vi "PicoScopeospaExampleStreamingQueue.vi"() -> ()   [LabVIEW 2010]
doc: "psospa Streaming example filling a single set of channel buffers at a time with LabVIEW queues."
uses:
  shared/PicoBuffers.ctl
  <vilib>/Waveform/DWDTOps.llb/DWDT Analog to Digital.vi
  PicoScopepsospaLib/PicoScopeospaDigitalChannelSettings.ctl
  PicoScopepsospaLib/PicoScopeospaAnalogChannelSettings.ctl
  shared/Buffer and Transfer Settings.ctl
panel:
  out "overflow":i16 format="%06b"
  in  "Channels":T1={"Channel A Settings "={"Enabled"=TRUE, "Coupling"=1, "Range"=8, "Analogue Offset"=0.0, "BandWidth"=0, "PROBE_RANGE_INFO"=0}, "Channel B Settings "={"Enabled"=FALSE, "Coupling"=1, "Range"=8, "Analogue Offset"=0.0, "BandWidth"=0, "PROBE_RANGE_INFO"=0}, "Channel C Settings "={"Enabled"=FALSE, "Coupling"=1, "Range"=8, "Analogue Offset"=0.0, "BandWidth"=0, "PROBE_RANGE_INFO"=0}, "Channel D Settings "={"Enabled"=FALSE, "Coupling"=1, "Range"=8, "Analogue Offset"=0.0, "BandWidth"=0, "PROBE_RANGE_INFO"=0}, "Channel E Settings "={"Enabled"=FALSE, "Coupling"=50, "Range"=5, "Analogue Offset"=0.0, "BandWidth"=0, "PROBE_RANGE_INFO"=0}, "Channel F Settings "={"Enabled"=FALSE, "Coupling"=50, "Range"=5, "Analogue Offset"=0.0, "BandWidth"=0, "PROBE_RANGE_INFO"=0}, "Channel G Settings "={"Enabled"=FALSE, "Coupling"=50, "Range"=5, "Analogue Offset"=0.0, "BandWidth"=0, "PROBE_RANGE_INFO"=0}, "Channel H Settings "={"Enabled"=FALSE, "Coupling"=50, "Range"=5, "Analogue Offset"=0.0, "BandWidth"=0, "PROBE_RANGE_INFO"=0}} {"Channel H Settings"."PROBE_RANGE_INFO" items=["PROBE_NONE_NV"=0, "X1_PROBE_NV"=1, "X10_PROBE_NV"=10]; "Channel H Settings"."BandWidth" items=["Full"=0, "100kHz"=100000, "20kHz"=200000, "1MHz"=1000000, "20MHz"=20000000, "25MHz"=25000000, "50MHz"=50000000, "200MHz"=200000000, "250MHz"=250000000, "500MHz"=500000000]; "Channel H Settings"."Range" items=["10mV"=0, "20mV"=1, "50mV"=2, "100mV"=3, "200mV"=4, "500mV"=5, "1V"=6, "2V"=7, "5V"=8, "10V"=9, "20V"=10, "50V"=11, "100V"=12, "200V"=13, "x10_Probe_100mV"=32, "x10_Probe_200mV"=33, "x10_Probe_500mV"=34, "x10_Probe_1V"=35, "x10_Probe_2V"=36, "x10_Probe_5V"=37, "x10_Probe_10V"=38, "x10_Probe_20V"=39, "x10_Probe_50V"=40, "x10_Probe_100V"=41, "x10_Probe_200V"=42, "x10_Probe_500V"=43, "CURRENT_CLAMP_60A_2A"=10500, "CURRENT_CLAMP_60A_5A"=10501, "CURRENT_CLAMP_60A_10A"=10502, "CURRENT_CLAMP_60A_20A"=10503, "CURRENT_CLAMP_60A_50A"=10504, "CURRENT_CLAMP_60A_60A"=10505, "CURRENT_CLAMP_60A_V2_0_5A"=10600, "CURRENT_CLAMP_60A_V2_1A"=10601, "CURRENT_CLAMP_60A_V2_2A"=10602, "CURRENT_CLAMP_60A_V2_5A"=10603, "CURRENT_CLAMP_60A_V2_10A"=10604, "CURRENT_CLAMP_60A_V2_20A"=10605, "CURRENT_CLAMP_60A_V2_50A"=10606, "CURRENT_CLAMP_60A_V2_60A"=10607, "RESISTANCE_LEAD_NEG5_TO_20OHM"=7000, "RESISTANCE_LEAD_NEG50_TO_200OHM"=7001, "RESISTANCE_LEAD_NEG500_TO_2KOHM"=7002, "RESISTANCE_LEAD_NEG5K_TO_20KOHM"=7003, "RESISTANCE_LEAD_NEG50K_TO_LEAD_200KOHM"=7004, "RESISTANCE_LEAD_NEG500K_TO_LEAD_2MOHM"=7005, "RESISTANCE_LEAD_DIODE_TEST"=7006, "HT_NEG3_TO_5KV"=8950, "HT_NEG3_TO_10KV"=8951, "HT_NEG5_TO_20KV"=8952, "HT_NEG5_TO_50KV"=8953, "HT_NEG5_TO_100KV"=8954, "HT_NEG3_TO_5KV_INVERTED"=8955, "HT_NEG3_TO_10KV_INVERTED"=8956, "HT_NEG5_TO_20KV_INVERTED"=8957, "HT_NEG5_TO_50KV_INVERTED"=8958, "HT_NEG5_TO_100KV_INVERTED"=8959, "TEMPERATURE_NEG50_TO_150DEGC"=9000, "PRESSURE_SENSOR_-100k-150k_PASCALS"=9100, "PRESSURE_SENSOR_-100k_TO_400k_PASCALS"=9101, "PRESSURE_SENSOR_-200k_TO_800k_PASCALS"=9102, "PRESSURE_SENSOR_-400k_TO_1600k_PASCALS"=9103, "PRESSURE_SENSOR_-400k_TO_3400k_PASCALS"=9104, "PRESSURE_SENSOR_-150k_TO_1350k_PASCALS"=9105]; "Channel H Settings"."Coupling" items=["AC"=0, "DC 1M Ohm"=1, "DC 50 Ohm"=50]; "Channel G Settings"."PROBE_RANGE_INFO" items=["PROBE_NONE_NV"=0, "X1_PROBE_NV"=1, "X10_PROBE_NV"=10]; "Channel G Settings"."BandWidth" items=["Full"=0, "100kHz"=100000, "20kHz"=200000, "1MHz"=1000000, "20MHz"=20000000, "25MHz"=25000000, "50MHz"=50000000, "200MHz"=200000000, "250MHz"=250000000, "500MHz"=500000000]; "Channel G Settings"."Range" items=["10mV"=0, "20mV"=1, "50mV"=2, "100mV"=3, "200mV"=4, "500mV"=5, "1V"=6, "2V"=7, "5V"=8, "10V"=9, "20V"=10, "50V"=11, "100V"=12, "200V"=13, "x10_Probe_100mV"=32, "x10_Probe_200mV"=33, "x10_Probe_500mV"=34, "x10_Probe_1V"=35, "x10_Probe_2V"=36, "x10_Probe_5V"=37, "x10_Probe_10V"=38, "x10_Probe_20V"=39, "x10_Probe_50V"=40, "x10_Probe_100V"=41, "x10_Probe_200V"=42, "x10_Probe_500V"=43, "CURRENT_CLAMP_60A_2A"=10500, "CURRENT_CLAMP_60A_5A"=10501, "CURRENT_CLAMP_60A_10A"=10502, "CURRENT_CLAMP_60A_20A"=10503, "CURRENT_CLAMP_60A_50A"=10504, "CURRENT_CLAMP_60A_60A"=10505, "CURRENT_CLAMP_60A_V2_0_5A"=10600, "CURRENT_CLAMP_60A_V2_1A"=10601, "CURRENT_CLAMP_60A_V2_2A"=10602, "CURRENT_CLAMP_60A_V2_5A"=10603, "CURRENT_CLAMP_60A_V2_10A"=10604, "CURRENT_CLAMP_60A_V2_20A"=10605, "CURRENT_CLAMP_60A_V2_50A"=10606, "CURRENT_CLAMP_60A_V2_60A"=10607, "RESISTANCE_LEAD_NEG5_TO_20OHM"=7000, "RESISTANCE_LEAD_NEG50_TO_200OHM"=7001, "RESISTANCE_LEAD_NEG500_TO_2KOHM"=7002, "RESISTANCE_LEAD_NEG5K_TO_20KOHM"=7003, "RESISTANCE_LEAD_NEG50K_TO_LEAD_200KOHM"=7004, "RESISTANCE_LEAD_NEG500K_TO_LEAD_2MOHM"=7005, "RESISTANCE_LEAD_DIODE_TEST"=7006, "HT_NEG3_TO_5KV"=8950, "HT_NEG3_TO_10KV"=8951, "HT_NEG5_TO_20KV"=8952, "HT_NEG5_TO_50KV"=8953, "HT_NEG5_TO_100KV"=8954, "HT_NEG3_TO_5KV_INVERTED"=8955, "HT_NEG3_TO_10KV_INVERTED"=8956, "HT_NEG5_TO_20KV_INVERTED"=8957, "HT_NEG5_TO_50KV_INVERTED"=8958, "HT_NEG5_TO_100KV_INVERTED"=8959, "TEMPERATURE_NEG50_TO_150DEGC"=9000, "PRESSURE_SENSOR_-100k-150k_PASCALS"=9100, "PRESSURE_SENSOR_-100k_TO_400k_PASCALS"=9101, "PRESSURE_SENSOR_-200k_TO_800k_PASCALS"=9102, "PRESSURE_SENSOR_-400k_TO_1600k_PASCALS"=9103, "PRESSURE_SENSOR_-400k_TO_3400k_PASCALS"=9104, "PRESSURE_SENSOR_-150k_TO_1350k_PASCALS"=9105]; "Channel G Settings"."Coupling" items=["AC"=0, "DC 1M Ohm"=1, "DC 50 Ohm"=50]; "Channel F Settings"."PROBE_RANGE_INFO" items=["PROBE_NONE_NV"=0, "X1_PROBE_NV"=1, "X10_PROBE_NV"=10]; "Channel F Settings"."BandWidth" items=["Full"=0, "100kHz"=100000, "20kHz"=200000, "1MHz"=1000000, "20MHz"=20000000, "25MHz"=25000000, "50MHz"=50000000, "200MHz"=200000000, "250MHz"=250000000, "500MHz"=500000000]; "Channel F Settings"."Range" items=["10mV"=0, "20mV"=1, "50mV"=2, "100mV"=3, "200mV"=4, "500mV"=5, "1V"=6, "2V"=7, "5V"=8, "10V"=9, "20V"=10, "50V"=11, "100V"=12, "200V"=13, "x10_Probe_100mV"=32, "x10_Probe_200mV"=33, "x10_Probe_500mV"=34, "x10_Probe_1V"=35, "x10_Probe_2V"=36, "x10_Probe_5V"=37, "x10_Probe_10V"=38, "x10_Probe_20V"=39, "x10_Probe_50V"=40, "x10_Probe_100V"=41, "x10_Probe_200V"=42, "x10_Probe_500V"=43, "CURRENT_CLAMP_60A_2A"=10500, "CURRENT_CLAMP_60A_5A"=10501, "CURRENT_CLAMP_60A_10A"=10502, "CURRENT_CLAMP_60A_20A"=10503, "CURRENT_CLAMP_60A_50A"=10504, "CURRENT_CLAMP_60A_60A"=10505, "CURRENT_CLAMP_60A_V2_0_5A"=10600, "CURRENT_CLAMP_60A_V2_1A"=10601, "CURRENT_CLAMP_60A_V2_2A"=10602, "CURRENT_CLAMP_60A_V2_5A"=10603, "CURRENT_CLAMP_60A_V2_10A"=10604, "CURRENT_CLAMP_60A_V2_20A"=10605, "CURRENT_CLAMP_60A_V2_50A"=10606, "CURRENT_CLAMP_60A_V2_60A"=10607, "RESISTANCE_LEAD_NEG5_TO_20OHM"=7000, "RESISTANCE_LEAD_NEG50_TO_200OHM"=7001, "RESISTANCE_LEAD_NEG500_TO_2KOHM"=7002, "RESISTANCE_LEAD_NEG5K_TO_20KOHM"=7003, "RESISTANCE_LEAD_NEG50K_TO_LEAD_200KOHM"=7004, "RESISTANCE_LEAD_NEG500K_TO_LEAD_2MOHM"=7005, "RESISTANCE_LEAD_DIODE_TEST"=7006, "HT_NEG3_TO_5KV"=8950, "HT_NEG3_TO_10KV"=8951, "HT_NEG5_TO_20KV"=8952, "HT_NEG5_TO_50KV"=8953, "HT_NEG5_TO_100KV"=8954, "HT_NEG3_TO_5KV_INVERTED"=8955, "HT_NEG3_TO_10KV_INVERTED"=8956, "HT_NEG5_TO_20KV_INVERTED"=8957, "HT_NEG5_TO_50KV_INVERTED"=8958, "HT_NEG5_TO_100KV_INVERTED"=8959, "TEMPERATURE_NEG50_TO_150DEGC"=9000, "PRESSURE_SENSOR_-100k-150k_PASCALS"=9100, "PRESSURE_SENSOR_-100k_TO_400k_PASCALS"=9101, "PRESSURE_SENSOR_-200k_TO_800k_PASCALS"=9102, "PRESSURE_SENSOR_-400k_TO_1600k_PASCALS"=9103, "PRESSURE_SENSOR_-400k_TO_3400k_PASCALS"=9104, "PRESSURE_SENSOR_-150k_TO_1350k_PASCALS"=9105]; "Channel F Settings"."Coupling" items=["AC"=0, "DC 1M Ohm"=1, "DC 50 Ohm"=50]; "Channel E Settings"."PROBE_RANGE_INFO" items=["PROBE_NONE_NV"=0, "X1_PROBE_NV"=1, "X10_PROBE_NV"=10]; "Channel E Settings"."BandWidth" items=["Full"=0, "100kHz"=100000, "20kHz"=200000, "1MHz"=1000000, "20MHz"=20000000, "25MHz"=25000000, "50MHz"=50000000, "200MHz"=200000000, "250MHz"=250000000, "500MHz"=500000000]; "Channel E Settings"."Range" items=["10mV"=0, "20mV"=1, "50mV"=2, "100mV"=3, "200mV"=4, "500mV"=5, "1V"=6, "2V"=7, "5V"=8, "10V"=9, "20V"=10, "50V"=11, "100V"=12, "200V"=13, "x10_Probe_100mV"=32, "x10_Probe_200mV"=33, "x10_Probe_500mV"=34, "x10_Probe_1V"=35, "x10_Probe_2V"=36, "x10_Probe_5V"=37, "x10_Probe_10V"=38, "x10_Probe_20V"=39, "x10_Probe_50V"=40, "x10_Probe_100V"=41, "x10_Probe_200V"=42, "x10_Probe_500V"=43, "CURRENT_CLAMP_60A_2A"=10500, "CURRENT_CLAMP_60A_5A"=10501, "CURRENT_CLAMP_60A_10A"=10502, "CURRENT_CLAMP_60A_20A"=10503, "CURRENT_CLAMP_60A_50A"=10504, "CURRENT_CLAMP_60A_60A"=10505, "CURRENT_CLAMP_60A_V2_0_5A"=10600, "CURRENT_CLAMP_60A_V2_1A"=10601, "CURRENT_CLAMP_60A_V2_2A"=10602, "CURRENT_CLAMP_60A_V2_5A"=10603, "CURRENT_CLAMP_60A_V2_10A"=10604, "CURRENT_CLAMP_60A_V2_20A"=10605, "CURRENT_CLAMP_60A_V2_50A"=10606, "CURRENT_CLAMP_60A_V2_60A"=10607, "RESISTANCE_LEAD_NEG5_TO_20OHM"=7000, "RESISTANCE_LEAD_NEG50_TO_200OHM"=7001, "RESISTANCE_LEAD_NEG500_TO_2KOHM"=7002, "RESISTANCE_LEAD_NEG5K_TO_20KOHM"=7003, "RESISTANCE_LEAD_NEG50K_TO_LEAD_200KOHM"=7004, "RESISTANCE_LEAD_NEG500K_TO_LEAD_2MOHM"=7005, "RESISTANCE_LEAD_DIODE_TEST"=7006, "HT_NEG3_TO_5KV"=8950, "HT_NEG3_TO_10KV"=8951, "HT_NEG5_TO_20KV"=8952, "HT_NEG5_TO_50KV"=8953, "HT_NEG5_TO_100KV"=8954, "HT_NEG3_TO_5KV_INVERTED"=8955, "HT_NEG3_TO_10KV_INVERTED"=8956, "HT_NEG5_TO_20KV_INVERTED"=8957, "HT_NEG5_TO_50KV_INVERTED"=8958, "HT_NEG5_TO_100KV_INVERTED"=8959, "TEMPERATURE_NEG50_TO_150DEGC"=9000, "PRESSURE_SENSOR_-100k-150k_PASCALS"=9100, "PRESSURE_SENSOR_-100k_TO_400k_PASCALS"=9101, "PRESSURE_SENSOR_-200k_TO_800k_PASCALS"=9102, "PRESSURE_SENSOR_-400k_TO_1600k_PASCALS"=9103, "PRESSURE_SENSOR_-400k_TO_3400k_PASCALS"=9104, "PRESSURE_SENSOR_-150k_TO_1350k_PASCALS"=9105]; "Channel E Settings"."Coupling" items=["AC"=0, "DC 1M Ohm"=1, "DC 50 Ohm"=50]; "Channel D Settings"."BandWidth" items=["Full"=0, "100kHz"=100000, "20kHz"=200000, "1MHz"=1000000, "20MHz"=20000000, "25MHz"=25000000, "50MHz"=50000000, "100MHz"=100000000, "200MHz"=200000000, "250MHz"=250000000, "350MHz"=350000000, "500MHz"=500000000]; "Channel D Settings"."PROBE_RANGE_INFO" items=["PROBE_NONE_NV"=0, "X1_PROBE_NV"=1, "X10_PROBE_NV"=10]; "Channel D Settings"."Range" items=["10mV", "20mV", "50mV", "100mV", "200mV", "500mV", "1V", "2V", "5V", "10V", "20V", "50V", "100V", "200V"]; "Channel D Settings"."Coupling" items=["AC"=0, "DC 1M Ohm"=1, "DC 50 Ohm"=50]; "Channel C Settings"."BandWidth" items=["Full"=0, "100kHz"=100000, "20kHz"=200000, "1MHz"=1000000, "20MHz"=20000000, "25MHz"=25000000, "50MHz"=50000000, "100MHz"=100000000, "200MHz"=200000000, "250MHz"=250000000, "350MHz"=350000000, "500MHz"=500000000]; "Channel C Settings"."PROBE_RANGE_INFO" items=["PROBE_NONE_NV"=0, "X1_PROBE_NV"=1, "X10_PROBE_NV"=10]; "Channel C Settings"."Range" items=["10mV", "20mV", "50mV", "100mV", "200mV", "500mV", "1V", "2V", "5V", "10V", "20V", "50V", "100V", "200V"]; "Channel C Settings"."Coupling" items=["AC"=0, "DC 1M Ohm"=1, "DC 50 Ohm"=50]; "Channel B Settings"."BandWidth" items=["Full"=0, "100kHz"=100000, "20kHz"=200000, "1MHz"=1000000, "20MHz"=20000000, "25MHz"=25000000, "50MHz"=50000000, "100MHz"=100000000, "200MHz"=200000000, "250MHz"=250000000, "350MHz"=350000000, "500MHz"=500000000]; "Channel B Settings"."PROBE_RANGE_INFO" items=["PROBE_NONE_NV"=0, "X1_PROBE_NV"=1, "X10_PROBE_NV"=10]; "Channel B Settings"."Range" items=["10mV", "20mV", "50mV", "100mV", "200mV", "500mV", "1V", "2V", "5V", "10V", "20V", "50V", "100V", "200V"]; "Channel B Settings"."Coupling" items=["AC"=0, "DC 1M Ohm"=1, "DC 50 Ohm"=50]; "Channel A Settings"."PROBE_RANGE_INFO" items=["PROBE_NONE_NV"=0, "X1_PROBE_NV"=1, "X10_PROBE_NV"=10]; "Channel A Settings"."Range" items=["10mV", "20mV", "50mV", "100mV", "200mV", "500mV", "1V", "2V", "5V", "10V", "20V", "50V", "100V", "200V"]; "Channel A Settings"."BandWidth" items=["Full"=0, "100kHz"=100000, "20kHz"=200000, "1MHz"=1000000, "20MHz"=20000000, "25MHz"=25000000, "50MHz"=50000000, "100MHz"=100000000, "200MHz"=200000000, "250MHz"=250000000, "350MHz"=350000000, "500MHz"=500000000]; "Channel A Settings"."Coupling" items=["AC"=0, "DC 1M Ohm"=1, "DC 50 Ohm"=50]}
  out "Triggered":bool
  out "triggerAt_":u64
  in  "Poll Delay %":dbl=1.0 format="%#_13g"
  in  "Poll Holdoff %":dbl=33.0 format="%#_13g"
  out "Port 0":digitalwaveform(graph)={"t0"=timestamp(0 s since 1904-01-01), "dt"=1.004800013071339e-06, "Y"={"transitions"=[], "data"=[]}}
  out "Analog Channels":cluster{i32, dbl, "Data":dbl[]}[](graph)
  in  "Write to file":bool
  out "Queue depth":i32(graph)
  out "queue depth":i32
  in  "Data file":path=path "PicoScopeospaExampleStreaming Data"
  out "Max ADC value":i16
  out "DownSample Interval (sec)":dbl=1.0000000130088963e-06 format="%#.5p"
  out "Chunk time":u32
  out "Elapsed time":dbl
  in  "Auto Stop":bool
  in  "Apply Settings":bool
  in  "Digital Channels":T2={"Port 0 Settings "={"Enabled"=FALSE, "Threshold Level (Volts)"=3.0}, "Port 1 Settings"={"Enabled"=FALSE, "Threshold Level (Volts)"=3.0}} {"Port 1 Settings"."Threshold Level (Volts)" format="%#_4p"; "Port 0 Settings"."Threshold Level (Volts)" format="%#_4p"}
  in  "No of Buffers":i32=2 min=2
  in  "Streaming Acquisition Settings":T3={"preTriggerSamples"=0, "postTriggerSamples"=100000, "Requested sampleInterval"=1.0, "sampleIntervalTimeUnits"=3} {"sampleIntervalTimeUnits" items=["femtoseconds", "picoseconds", "nanoseconds", "microseconds", "millseconds", "seconds"]; "postTriggerSamples" format="%_6p"; "preTriggerSamples" format="%_6p"}
  in  "Buffer and Transfer Settings":T4={"startIndex"=0, "Samples"=100000, "Down Sample Ratio"=1, "Down-Sample Mode"=2147483648} {"Down-Sample Mode" items=["RAW none"=2147483648, "None"=0, "Aggregate"=1, "Decimate"=2, "Average"=4]; "Down Sample Ratio" step=1; "Samples" format="%_6p"}
  in  "Trigger Settings":T5={"Trigger Enabled"=FALSE, "Trigger Threshold (Volts)"=0.0, "Trigger Direction"=2, "Trigger Delay (samples)"=0, "Auto Trigger Time (us)"=100000, "Trigger Source"=0} {"Trigger Source" items=["Channel A"=0, "Channel B"=1, "Channel C"=2, "Channel D"=3, "Channel E"=4, "Channel F"=5, "Channel G"=6, "Channel H"=7, "Port 0"=128, "Port 1"=129, "Trigger AUX"=1001]; "Trigger Direction" items=["Rising"=2, "Falling"=3]; "Trigger Threshold (Volts)" format="%#_6p"}
  in  "stop":bool
  out "Device Info":T6
  out "Pico ospa Units":string
  in  "Resolution":u32(ring)=10 items=["8-bit"=0, "12-bit"=1, "14-bit"=2, "15-bit"=3, "16-bit"=4, "10-bit"=10]
  in  "Serial Number":string
  in  "Use Serial Number":bool
  in  "error in (no error)":errorcluster
  # "LSB ChA"
  # "D8-D15"
  # "DO-D7"
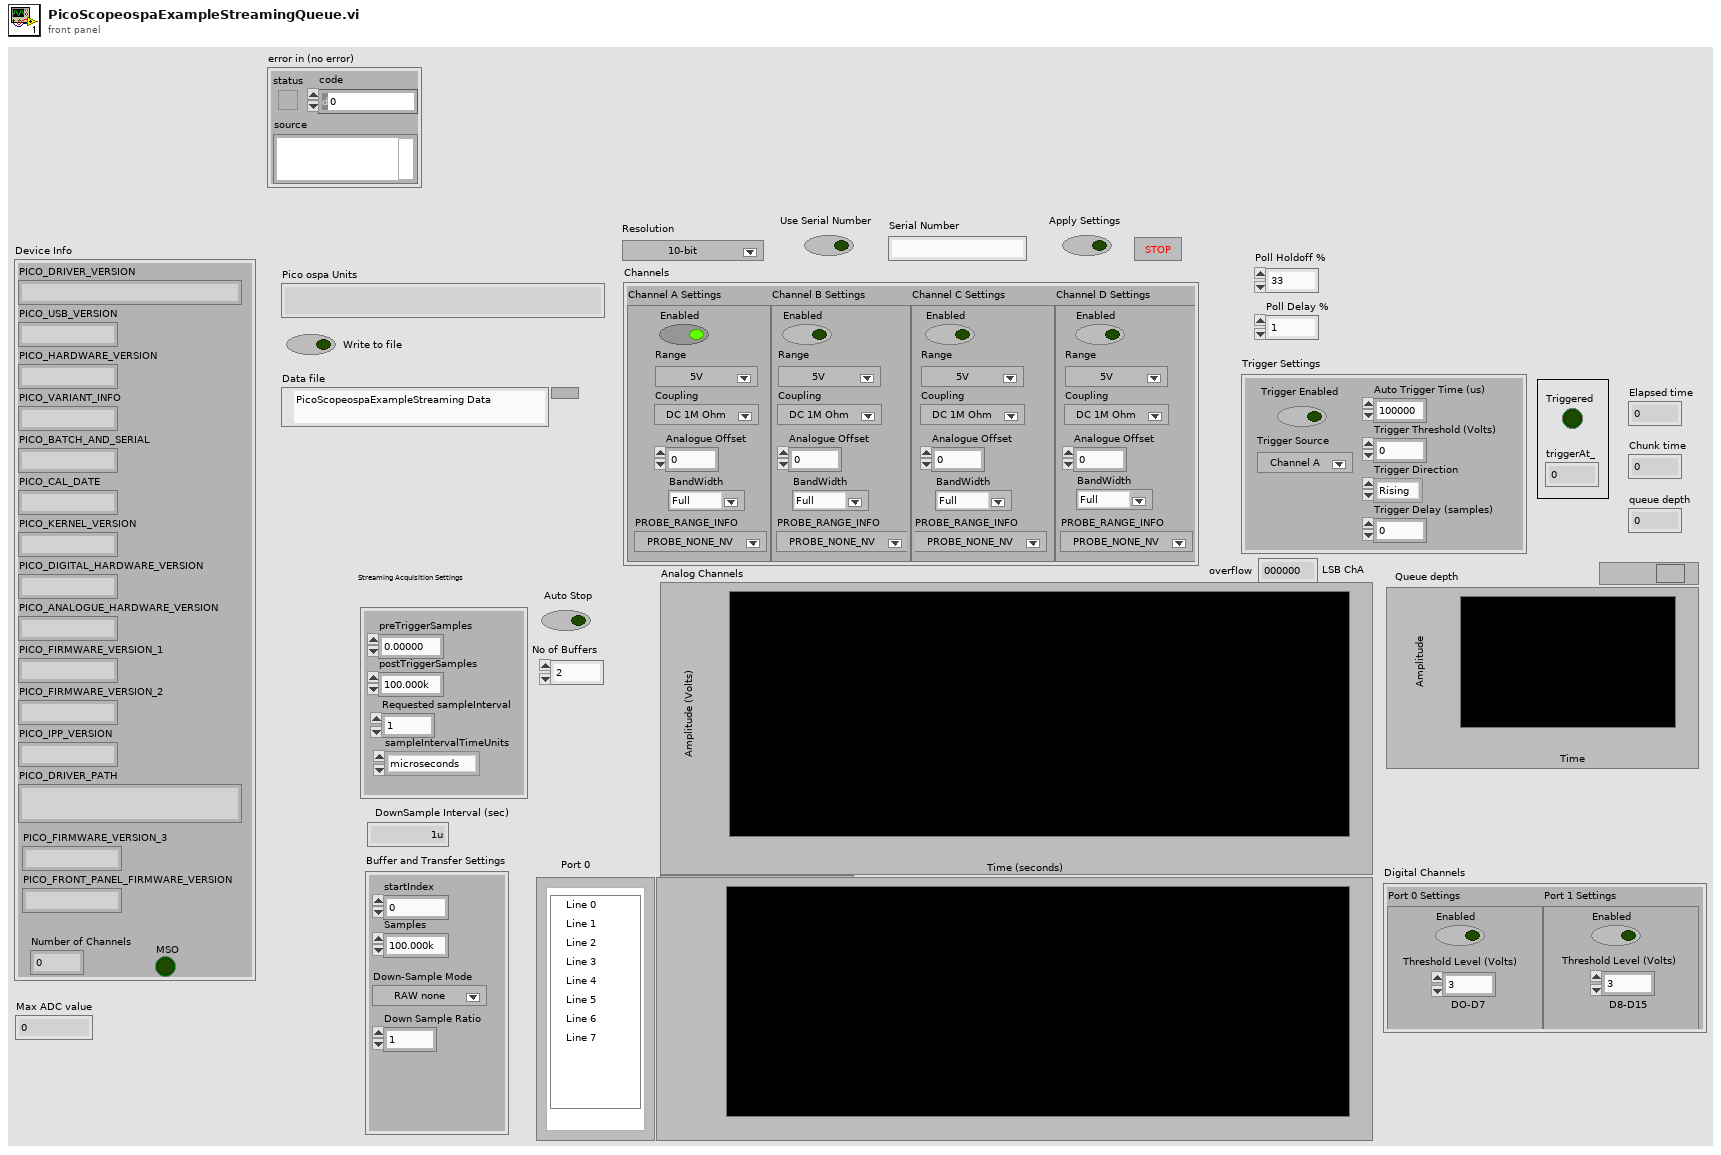
[diagram p1: front panel]
types:
  T1 = typedef "PicoScopeospaAnalogChannelSettings.ctl" = cluster{"Channel A Settings ":cluster{"Enabled":bool, "Coupling":i16, "Range":u16, "Analogue Offset":dbl, "BandWidth":u32, "PROBE_RANGE_INFO":u32}, "Channel B Settings ":cluster{"Enabled":bool, "Coupling":i16, "Range":u16, "Analogue Offset":dbl, "BandWidth":u32, "PROBE_RANGE_INFO":u32}, "Channel C Settings ":cluster{"Enabled":bool, "Coupling":i16, "Range":u16, "Analogue Offset":dbl, "BandWidth":u32, "PROBE_RANGE_INFO":u32}, "Channel D Settings ":cluster{"Enabled":bool, "Coupling":i16, "Range":u16, "Analogue Offset":dbl, "BandWidth":u32, "PROBE_RANGE_INFO":u32}, "Channel E Settings ":cluster{"Enabled":bool, "Coupling":i16, "Range":u16, "Analogue Offset":dbl, "BandWidth":u32, "PROBE_RANGE_INFO":u32}, "Channel F Settings ":cluster{"Enabled":bool, "Coupling":i16, "Range":u16, "Analogue Offset":dbl, "BandWidth":u32, "PROBE_RANGE_INFO":u32}, "Channel G Settings ":cluster{"Enabled":bool, "Coupling":i16, "Range":u16, "Analogue Offset":dbl, "BandWidth":u32, "PROBE_RANGE_INFO":u32}, "Channel H Settings ":cluster{"Enabled":bool, "Coupling":i16, "Range":u16, "Analogue Offset":dbl, "BandWidth":u32, "PROBE_RANGE_INFO":u32}}
  T2 = typedef "PicoScopeospaDigitalChannelSettings.ctl" = cluster{"Port 0 Settings ":cluster{"Enabled":bool, "Threshold Level (Volts)":dbl}, "Port 1 Settings":cluster{"Enabled":bool, "Threshold Level (Volts)":dbl}}
  T3 = cluster{"preTriggerSamples":u64, "postTriggerSamples":u64, "Requested sampleInterval":dbl, "sampleIntervalTimeUnits":u32}
  T4 = typedef "Buffer and Transfer Settings.ctl" = cluster{"startIndex":u64, "Samples":u64, "Down Sample Ratio":u64, "Down-Sample Mode":u32}
  T5 = cluster{"Trigger Enabled":bool, "Trigger Threshold (Volts)":dbl, "Trigger Direction":u16, "Trigger Delay (samples)":u64, "Auto Trigger Time (us)":u32, "Trigger Source":u32}
  T6 = cluster{"PICO_DRIVER_VERSION":string, "PICO_USB_VERSION":string, "PICO_HARDWARE_VERSION":string, "PICO_VARIANT_INFO":string, "PICO_BATCH_AND_SERIAL":string, "PICO_CAL_DATE":string, "PICO_KERNEL_VERSION":string, "PICO_DIGITAL_HARDWARE_VERSION":string, "PICO_ANALOGUE_HARDWARE_VERSION":string, "PICO_FIRMWARE_VERSION_1":string, "PICO_FIRMWARE_VERSION_2":string, "PICO_IPP_VERSION":string, "PICO_DRIVER_PATH":string, "PICO_FIRMWARE_VERSION_3":string, "PICO_FRONT_PANEL_FIRMWARE_VERSION":string, "Number of Channels":i16, "MSO":bool}
  T7 = typedef "PicoBuffers.ctl" = cluster{"Max Buffer Pointers":u64[][][], "Min Buffer Pointers":u64[][][], "StreamingDataInfo":cluster{"Channel":u32, "Down-Sample Mode":u32, "PICO_DATA_TYPE":enum32{"PICO_INT8_T", "PICO_INT16_T", "PICO_INT32_T", "PICO_UINT32_T", "PICO_INT64_T", ""}, "Samples":i32, "bufferIndex":u64, "startIndex":i32, "overflow":i16}[][]}
  T8 = enum16{"open", "open or create", "create or replace", "create", "open (read-only)"}
  T9 = cluster{"sampleInterval":dbl, "sampleIntervalTimeUnits":u32}
  T10 = cluster{"triggerAt":u64, "triggered":bool, "autoStop":bool}
  T11 = cluster{"Channel A Buffer":i16[], "Channel B Buffer":i16[], "Channel C Buffer":i16[], "Channel D Buffer":i16[], "Channel E Buffer":i16[], "Channel F Buffer":i16[], "Channel G Buffer":i16[], "Channel H Buffer":i16[], "Port 0 Buffer":i16[], "Port 1 Buffer":i16[]}
  T12 = cluster{"Channel":u32, "Down-Sample Mode":u32, "PICO_DATA_TYPE":enum32{"PICO_INT8_T", "PICO_INT16_T", "PICO_INT32_T", "PICO_UINT32_T", "PICO_INT64_T", ""}, "Samples":i32, "bufferIndex":u64, "startIndex":i32, "overflow":i16}[][]
  T13 = cluster{"Channel":u32, "Down-Sample Mode":u32, "PICO_DATA_TYPE":enum32{"PICO_INT8_T", "PICO_INT16_T", "PICO_INT32_T", "PICO_UINT32_T", "PICO_INT64_T", ""}, "Samples":i32, "bufferIndex":u64, "startIndex":i32, "overflow":i16}[]
  T14 = cluster{"Channel":u32, "Down-Sample Mode":u32, "PICO_DATA_TYPE":enum32{"PICO_INT8_T", "PICO_INT16_T", "PICO_INT32_T", "PICO_UINT32_T", "PICO_INT64_T", ""}, "Samples":i32, "bufferIndex":u64, "startIndex":i32, "overflow":i16}
  T15 = cluster{i32, "DownSample Interval (sec)":dbl, "Data":dbl[]}
  T16 = cluster{i32, "DownSample Interval (sec)":dbl, "Data":dbl[]}[]
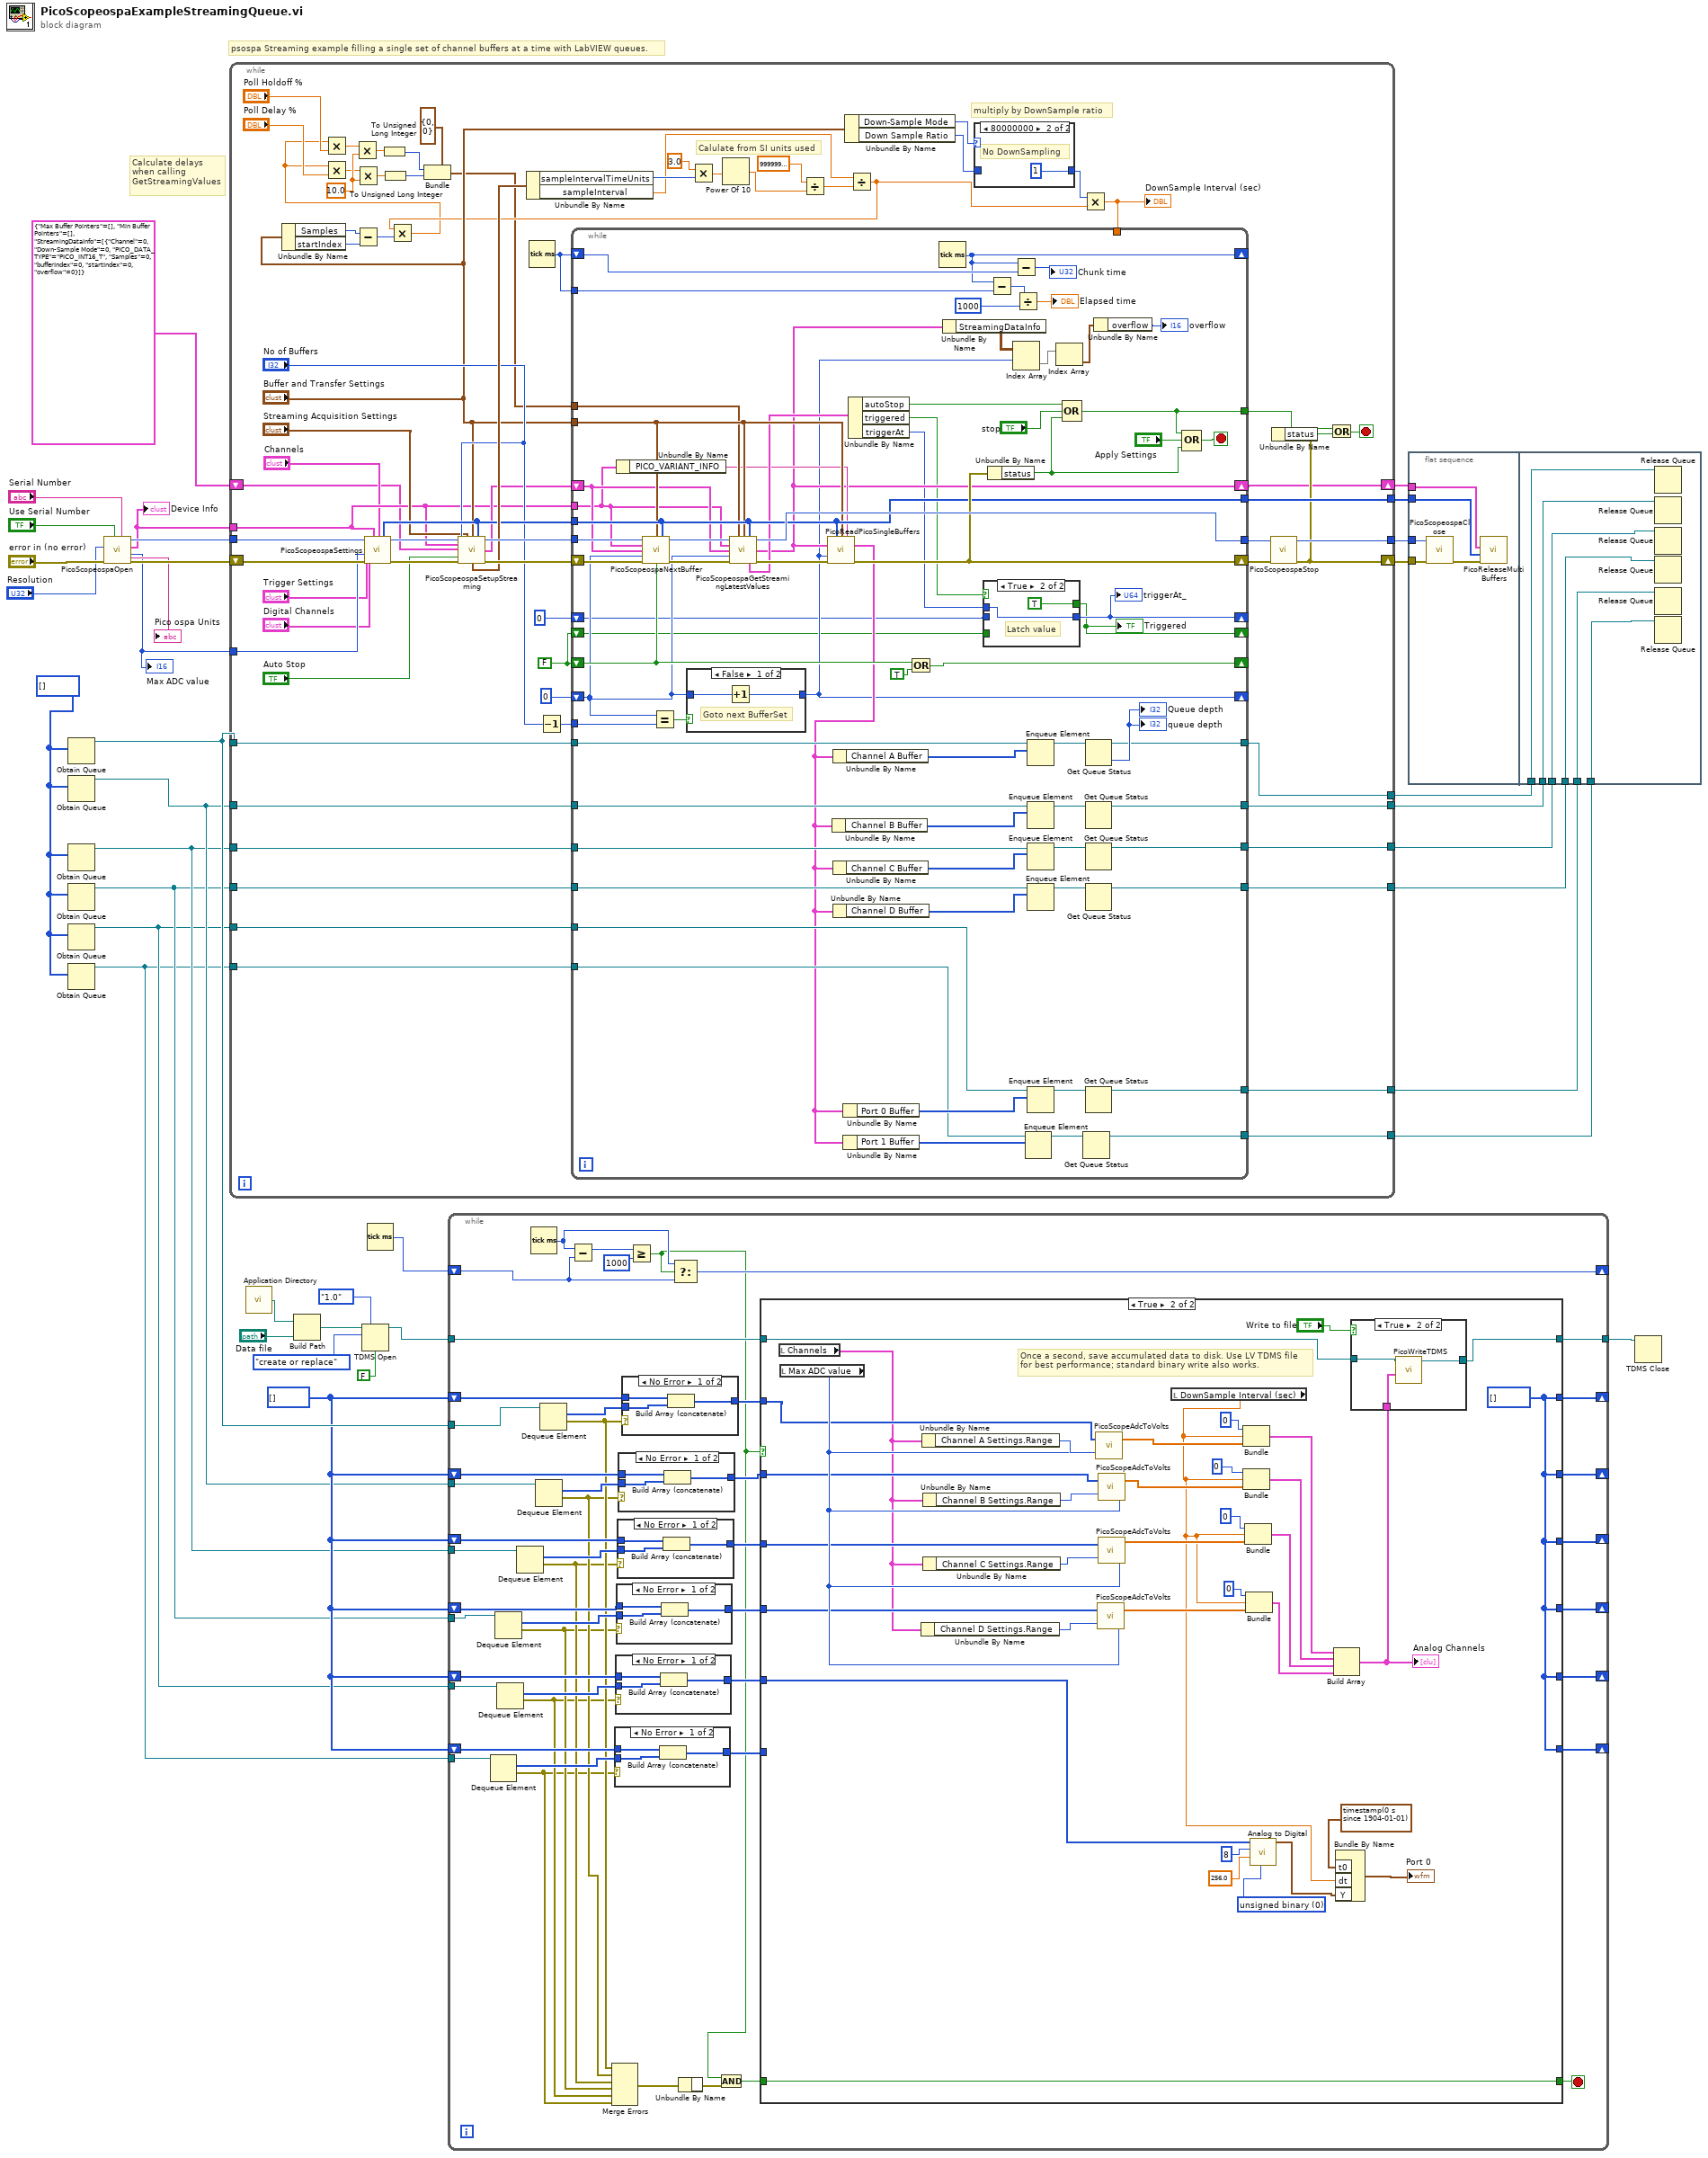
[diagram p0: block diagram]
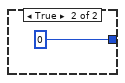
[diagram p11: hidden frame]
diagram:
  w12 = i16[] [] ("History Data")
  w13 = i16[] [] ("History Data")
  # "Calculate delays\nwhen calling\nGetStreamingValues"
  # "psospa Streaming example filling a single set of channel buffers at a time with LabVIEW queues."
  n1 = Obtain Queue(element data type=w12) -> (queue out=w14:refnum<queue>)  [unwired: 4 in, 2 out]
  n2 = Obtain Queue(element data type=w12) -> (queue out=w11:refnum<queue>)  [unwired: 4 in, 2 out]
  n3 = Obtain Queue(element data type=w12) -> (queue out=w10:refnum<queue>)  [unwired: 4 in, 2 out]
  n4 = Obtain Queue(element data type=w12) -> (queue out=w9:refnum<queue>)  [unwired: 4 in, 2 out]
  n5 = Obtain Queue(element data type=w12) -> (queue out=w8:refnum<queue>)  [unwired: 4 in, 2 out]
  n6 = Obtain Queue(element data type=w12) -> (queue out=w7:refnum<queue>)  [unwired: 4 in, 2 out]
  n7 = call "PicoScopeospaOpen.vi"("Serial Number"="Serial Number", "Use Serial Number"="Use Serial Number", "error in (no error)"="error in (no error)", "Resolution"="Resolution") -> ("error out"=w33:errorcluster, "Max ADC value"=w20:i16, "Device Info"=w30:T6, "handle out"=w34:i16, "psospa Units"=→"Pico ospa Units":string)  [unwired: 2 in, 1 out]
  "Device Info" <- w30
  "Max ADC value" <- w20
  n8 = while {
    tunnel: w34 -> [w109]
    tunnel: [w80] -> w17
    tunnel: w30 -> [w45]
    tunnel: w20 -> [w107]
    tunnel: [w92] -> w19
    shift-right: [w79] -> w18
    shift-left: w33 -> [w108]
    tunnel: w14 -> [w74]
    tunnel: w11 -> [w73]
    tunnel: [w72] -> w16
    tunnel: [w71] -> w15
    tunnel: w10 -> [w70]
    tunnel: w9 -> [w69]
    tunnel: w8 -> [w68]
    tunnel: w7 -> [w67]
    tunnel: [w66] -> w6
    tunnel: [w65] -> w5
    tunnel: [w64] -> w4
    tunnel: [w42] -> w3
    shift-right: [w38] -> w1
    shift-left: T7 {"Max Buffer Pointers"=[], "Min Buffer Pointers"=[], "StreamingDataInfo"=[[{"Channel"=0, "Down-Sample Mode"=0, "PICO_DATA_TYPE"=enum."PICO_INT16_T", "Samples"=0, "bufferIndex"=0, "startIndex"=0, "overflow"=0}]]} ("Data Pointers") -> [w39]
    stop <- w87 stop-if-true
    w55 = 10.0 ("y")
    w40 = FALSE ("SetDataBuffer0")
    # "Calulate from SI units used"
    # "multiply by DownSample ratio"
    n9 = Unbundle By Name("Buffer and Transfer Settings") -> ("Samples"=w47:u64, "startIndex"=w48:u64)
    n10 = Subtract(x=w47, y=w48) -> (x-y=w46:u64)
    n11 = call "PicoScopeospaSettings.vi"("handle in"=w109, "Device Info"=w45, "Channels"="Channels", "Max ADC value"=w107, "error in (no error)"=w108, "Trigger Settings"="Trigger Settings", "Digital Channels"="Digital Channels") -> ("Enabled array"=w90:i16[], "handle out"=w103:i16, "error out"=w104:errorcluster)  [unwired: 6 in]
    n12 = call "PicoScopeospaSetupStreaming.vi"("handle in"=w103, "Streaming Acquisition Settings"="Streaming Acquisition Settings", "Buffer and Transfer Settings"="Buffer and Transfer Settings", "enabled array"=w90, "Device Info"=w45, "Data Pointers In"=w39, "Number of Buffers"="No of Buffers", "error in (no error)"=w104, "Auto Stop"="Auto Stop") -> ("handle out"=w96:i16, "Data Pointers"=w85:T7, "Actual sampleInterval"=w94:T9, "error out"=w95:errorcluster)  [unwired: 3 in]
    n13 = Unbundle By Name(w94) -> ("sampleIntervalTimeUnits"=w99:u32, "sampleInterval"=w93:dbl)
    n14 = Tick Count (ms)() -> (millisecond timer value=w44:u32)
    n15 = Decrement(x="No of Buffers") -> (x-1=w75:i32)
    n16 = Multiply(x=3.0, y=w99) -> (x*y=w100:dbl)
    n17 = Power Of 10(x=w100) -> (10^x=w98:dbl)
    n18 = Divide(x=sgl 1000000000000000.0 ("y"), y=w98) -> (x/y=w97:dbl)
    n19 = Unbundle By Name("Buffer and Transfer Settings") -> ("Down-Sample Mode"=w81:u32, "Down Sample Ratio"=w82:u64)
    n20 = Divide(x=w93, y=w97) -> (x/y=w61:dbl)
    n21 = Multiply(x=w61, y=w46) -> (x*y=w49:dbl)
    n22 = Multiply(x=w49, y="Poll Holdoff %") -> (x*y=w53:dbl)
    n23 = Multiply(x=w49, y="Poll Delay %") -> (x*y=w54:dbl)
    n24 = Multiply(x=w53, y=w55) -> (x*y=w58:dbl)
    n25 = Multiply(x=w54, y=w55) -> (x*y=w59:dbl)
    n26 = To Unsigned Long Integer(number=w58) -> (unsigned 32bit integer=w56:u32)
    n27 = To Unsigned Long Integer(number=w59) -> (unsigned 32bit integer=w57:u32)
    n28 = Bundle(cluster=cluster{u32, u32} {0, 0}, w56, w57) -> (w60:cluster{u32, u32})
    n29 = case shown="80000000" w81 {
      tunnel: [w188 u64 1 ("Down Sample Ratio")] -> w105
      tunnel: w82 -> [w188 _]
      frame Default {
      }
      frame -2147483648 {
        # "No DownSampling"
      }
    }
    n30 = Multiply(x=w105, y=w61) -> (x*y=w63:dbl)
    "DownSample Interval (sec)" <- w63
    n31 = while {
      tunnel: w63 -> [_]
      tunnel: "Buffer and Transfer Settings" -> [w165]
      tunnel: w96 -> [w172]
      tunnel: w90 -> [w166]
      tunnel: [w168] -> w77
      shift-right: [w167] -> w78
      shift-left: w95 -> [w173]
      shift-right: [w179] -> _
      shift-left: w40 -> [w164]
      tunnel: [w166] -> w92
      tunnel: [w175] -> w88
      tunnel: w45 -> [w130]
      tunnel: w60 -> [w132]
      shift-right: [w116] -> _
      shift-left: 0 ("No of Buffers") -> [w161]
      shift-right: [w119] -> w38
      shift-left: w85 -> [w163]
      tunnel: w75 -> [w159]
      shift-right: [w153] -> _
      shift-left: w44 -> [w154]
      tunnel: w74 -> [w149]
      tunnel: w73 -> [w148]
      tunnel: [w147] -> w72
      tunnel: [w146] -> w71
      tunnel: w70 -> [w143]
      tunnel: w69 -> [w142]
      tunnel: w68 -> [w128]
      tunnel: w67 -> [w125]
      tunnel: [w140] -> w66
      tunnel: [w139] -> w65
      tunnel: [w138] -> w64
      tunnel: w44 -> [w129]
      tunnel: [w126] -> w42
      shift-right: [w114] -> _
      shift-left: u64 0 ("triggerAt") -> [w115]
      shift-right: [w112] -> _
      shift-left: w40 -> [w113]
      stop <- w178 stop-if-true
      n32 = Unbundle By Name(w130) -> ("PICO_VARIANT_INFO"=w131:string)
      n33 = call "PicoScopeospaNextBuffer.vi"("handle in"=w172, "Buffer and Transfer Settings"=w165, "enabled array"=w166, "Device Info"=w130, "Data Pointers In"=w163, "Buffer Number"=w161, "error in (no error)"=w173, "LoopFlag"=w164) -> ("handle out"=w169:i16, "error out"=w171:errorcluster)  [unwired: 6 in]
      n34 = Equal?(x=w161, y=w159) -> (x = y?=w162:bool)
      n35 = case shown="False" w162 {
        tunnel: w161 -> [w186 _]
        tunnel: [w185 0] -> w116
        frame False {
          # "Goto next BufferSet"
          n36 = Increment(x=w186) -> (x+1=w185:i32)
        }
        frame True {
        }
      }
      n37 = call "PicoScopeospaGetStreamingLatestValues.vi"("handle in"=w169, "Polling Delays ms"=w132, "Buffer and Transfer Settings"=w165, "enabled array"=w166, "Device Info"=w130, "Data Pointers In"=w163, "Buffer number"=w161, "error in (no error)"=w171) -> ("handle out"=w168:i16, "Data Pointers Out"=w119:T7, "tPicoStreamingDataTriggerInfo"=w160:T10, "error out"=w170:errorcluster)  [unwired: 4 in]
      n38 = call "PicoReadPicoSingleBuffers.vi"("enabled array"=w166, "Buffer and Transfer Settings"=w165, "Variant"=w131, "Data Pointers"=w119, "Buffer Number"=w116, "error in (no error)"=w170) -> ("MaxBuffers (Max or non-aggregated)"=w124:T11, "error out"=w167:errorcluster)  [unwired: 7 in, 1 out]
      n39 = Unbundle By Name(w124) -> ("Channel B Buffer"=w137:i16[])
      n40 = Unbundle By Name(w124) -> ("Channel A Buffer"=w133:i16[])
      n41 = Unbundle By Name(w124) -> ("Channel C Buffer"=w136:i16[])
      n42 = Unbundle By Name(w124) -> ("Channel D Buffer"=w135:i16[])
      n43 = Unbundle By Name(w124) -> ("Port 0 Buffer"=w134:i16[])
      n44 = Unbundle By Name(w124) -> ("Port 1 Buffer"=w123:i16[])
      n45 = Unbundle By Name(w160) -> ("autoStop"=w122:bool, "triggered"=w111:bool, "triggerAt"=w110:u64)
      n46 = Or(x=w164, y=TRUE) -> (x .or. y?=w179:bool)
      n47 = Tick Count (ms)() -> (millisecond timer value=w153:u32)
      n48 = Unbundle By Name(w119) -> ("StreamingDataInfo"=w118:T12)
      n49 = case shown="True" w111 {
        tunnel: [w182 TRUE] -> w112
        tunnel: [w181 w183] -> w114
        tunnel: w115 -> [w181 _]
        tunnel: w110 -> [_ w183]
        tunnel: w113 -> [w182 _]
        frame False {
        }
        frame True {
          # "Latch value"
        }
      }
      "Triggered" <- w112
      "triggerAt_" <- w114
      n50 = Unbundle By Name(w167) -> ("status"=w174:bool)
      n51 = Subtract(x=w153, y=w129) -> (x-y=w156:u32)
      n52 = Subtract(x=w153, y=w154) -> (x-y=→"Chunk time":u32)
      n53 = Index Array(array=w118, index (row)=w116) -> (element=w117:T13)  [unwired: 1 in]
      n54 = Divide(x=w156, y=u32 1000) -> (x/y=→"Elapsed time":dbl)
      n55 = Enqueue Element(queue=w125, element=w123) -> (queue out=w127:refnum<queue>)  [unwired: 2 in, 2 out]
      n56 = Enqueue Element(queue=w149, element=w133) -> (queue out=w151:refnum<queue>)  [unwired: 2 in, 2 out]
      n57 = Enqueue Element(queue=w148, element=w137) -> (queue out=w150:refnum<queue>)  [unwired: 2 in, 2 out]
      n58 = Enqueue Element(queue=w143, element=w136) -> (queue out=w145:refnum<queue>)  [unwired: 2 in, 2 out]
      n59 = Enqueue Element(queue=w142, element=w135) -> (queue out=w144:refnum<queue>)  [unwired: 2 in, 2 out]
      n60 = Enqueue Element(queue=w128, element=w134) -> (queue out=w141:refnum<queue>)  [unwired: 2 in, 2 out]
      n61 = Index Array(array=w117) -> (element=w121:T14)  [unwired: 1 in]
      n62 = Compound Arithmetic op=OR(w122, "stop", w174) -> (w175:bool)
      n63 = Get Queue Status(queue=w127) -> (queue out=w126:refnum<queue>)  [unwired: 2 in, 7 out]
      n64 = Get Queue Status(queue=w151) -> (queue out=w147:refnum<queue>, # elements in queue=→"queue depth" →"Queue depth":i32)  [unwired: 2 in, 6 out]
      n65 = Get Queue Status(queue=w150) -> (queue out=w146:refnum<queue>)  [unwired: 2 in, 7 out]
      n66 = Get Queue Status(queue=w145) -> (queue out=w140:refnum<queue>)  [unwired: 2 in, 7 out]
      n67 = Get Queue Status(queue=w144) -> (queue out=w139:refnum<queue>)  [unwired: 2 in, 7 out]
      n68 = Get Queue Status(queue=w141) -> (queue out=w138:refnum<queue>)  [unwired: 2 in, 7 out]
      n69 = Unbundle By Name(w121) -> ("overflow"=→"overflow":i16)
      n70 = Compound Arithmetic op=OR(w175, "Apply Settings", w174) -> (w178:bool)
    }
    n71 = call "PicoScopeospaStop.vi"("error in (no error)"=w78, "handle in"=w77) -> ("error out"=w79:errorcluster, "handle out"=w80:i16)  [unwired: 8 in]
    n72 = Unbundle By Name(w79) -> ("status"=w89:bool)
    n73 = Or(x=w88, y=w89) -> (x .or. y?=w87:bool)
  }
  n74 = call <vilib>:"Application Directory.vi"() -> ("Application Directory"=w21:path)
  n75 = Build Path(base path=w21, name or relative path="Data file") -> (appended path=w22:path)
  n76 = TDMS Open(6:FALSE ("disable buffering? (T)"), 7:enum16{"1.0", "2.0"}."1.0" ("file format version (2.0)"), 10:T8."create or replace" ("operation (0:open)"), 11:w22) -> (3:w27:refnum<k34>)  [unwired: 2 in, 1 out]
  n77 = Tick Count (ms)() -> (millisecond timer value=w29:u32)
  n78 = while {
    tunnel: w14 -> [w236]
    shift-right: [w228] -> _
    shift-left: w13 -> [w235]
    shift-right: [w230] -> _
    shift-left: w29 -> [w231]
    tunnel: w27 -> [w227]
    tunnel: [w226] -> w26
    shift-right: [w218] -> _
    shift-left: w13 -> [w219]
    shift-right: [w215] -> _
    shift-left: w13 -> [w216]
    shift-right: [w210] -> _
    shift-left: w13 -> [w213]
    shift-right: [w209] -> _
    shift-left: w13 -> [w212]
    shift-right: [w208] -> _
    shift-left: w13 -> [w211]
    tunnel: w11 -> [w198]
    tunnel: w10 -> [w197]
    tunnel: w9 -> [w196]
    tunnel: w8 -> [w195]
    tunnel: w7 -> [w194]
    stop <- w225 stop-if-true
    n79 = Dequeue Element(queue=w194) -> (element=w220:i16[], error out=w199:errorcluster)  [unwired: 2 in, 2 out]
    n80 = Dequeue Element(queue=w196) -> (element=w222:i16[], error out=w201:errorcluster)  [unwired: 2 in, 2 out]
    n81 = Dequeue Element(queue=w195) -> (element=w221:i16[], error out=w200:errorcluster)  [unwired: 2 in, 2 out]
    n82 = Dequeue Element(queue=w197) -> (element=w223:i16[], error out=w202:errorcluster)  [unwired: 2 in, 2 out]
    n83 = Tick Count (ms)() -> (millisecond timer value=w232:u32)
    n84 = Dequeue Element(queue=w198) -> (element=w224:i16[], error out=w203:errorcluster)  [unwired: 2 in, 2 out]
    n85 = Dequeue Element(queue=w236) -> (element=w237:i16[], error out=w204:errorcluster)  [unwired: 2 in, 2 out]
    n86 = Subtract(x=w232, y=w231) -> (x-y=w234:u32)
    n87 = Merge Errors(w204, w203, w202, w201, w200, w199) -> (w193:errorcluster)
    n88 = case shown="No Error" w199 {
      tunnel: w211 -> [w240 w241]
      tunnel: [w239 w241] -> w205
      tunnel: w220 -> [w238 _]
      frame No Error {
        n89 = Build Array (concatenate)(w240, w238) -> (w239:i16[])
      }
      frame Error {
      }
    }
    n90 = case shown="No Error" w200 {
      tunnel: w212 -> [w244 w245]
      tunnel: [w243 w245] -> w206
      tunnel: w221 -> [w242 _]
      frame No Error {
        n91 = Build Array (concatenate)(w244, w242) -> (w243:i16[])
      }
      frame Error {
      }
    }
    n92 = case shown="No Error" w201 {
      tunnel: w213 -> [w248 w249]
      tunnel: [w247 w249] -> w207
      tunnel: w222 -> [w246 _]
      frame No Error {
        n93 = Build Array (concatenate)(w248, w246) -> (w247:i16[])
      }
      frame Error {
      }
    }
    n94 = case shown="No Error" w202 {
      tunnel: w216 -> [w252 w253]
      tunnel: [w251 w253] -> w214
      tunnel: w223 -> [w250 _]
      frame No Error {
        n95 = Build Array (concatenate)(w252, w250) -> (w251:i16[])
      }
      frame Error {
      }
    }
    n96 = case shown="No Error" w203 {
      tunnel: w219 -> [w256 w257]
      tunnel: [w255 w257] -> w217
      tunnel: w224 -> [w254 _]
      frame No Error {
        n97 = Build Array (concatenate)(w256, w254) -> (w255:i16[])
      }
      frame Error {
      }
    }
    n98 = case shown="No Error" w204 {
      tunnel: w235 -> [w308 w309]
      tunnel: [w307 w309] -> w229
      tunnel: w237 -> [w306 _]
      frame No Error {
        n99 = Build Array (concatenate)(w308, w306) -> (w307:i16[])
      }
      frame Error {
      }
    }
    n100 = Greater Or Equal?(x=w234, y=u32 1000) -> (x >= y?=w192:bool)
    n101 = Select(t=w232, s=w192, f=w231) -> (s? t:f=w230:u32)
    n102 = And(x=w192) -> (y=w190:errorcluster, x .and. y?=w191:bool)
    n103 = Unbundle By Name(w193, w190) -> ()
    n104 = case shown="True" w192 {
      tunnel: w229 -> [w265 w277]
      tunnel: [w265 w274] -> w228
      tunnel: w227 -> [w264 w269]
      tunnel: [w264 w268] -> w226
      tunnel: [w263 w301] -> w225
      tunnel: w191 -> [w263 w301]
      tunnel: [w262 w274] -> w218
      tunnel: w217 -> [w262 w276]
      tunnel: [w261 w274] -> w215
      tunnel: w214 -> [w261 w275]
      tunnel: [w260 w274] -> w210
      tunnel: [w259 w274] -> w209
      tunnel: [w258 w274] -> w208
      tunnel: w207 -> [w260 w273]
      tunnel: w206 -> [w259 w270]
      tunnel: w205 -> [w258 _]
      frame False {
      }
      frame True {
        w287 = u16 0 items=["unsigned binary", "offset binary", "2's complement"] ("data format (offset binary)")
        w274 = i16[] [] ("History Data")
        # "Once a second, save accumulated data to disk. Use LV TDMS file\nfor best performance; standard binary write also works."
        n105 = local read "Channels"() -> (w272:T1)
        n106 = local read "Max ADC value"() -> (w278:i16)
        n107 = Unbundle By Name(w272) -> ("Channel D Settings.Range"=w293:u16)
        n108 = Unbundle By Name(w272) -> ("Channel A Settings.Range"=w300:u16)
        n109 = Unbundle By Name(w272) -> ("Channel B Settings.Range"=w299:u16)
        n110 = Unbundle By Name(w272) -> ("Channel C Settings.Range"=w294:u16)
        n111 = call "PicoScopeAdcToVolts.vi"("Max_adc"=w278, "Range Index"=w300, "Data"=w277) -> ("Data"=w298:dbl[])
        n112 = call "PicoScopeAdcToVolts.vi"("Max_adc"=w278, "Range Index"=w293, "Data"=w273) -> ("Data"=w291:dbl[])
        n113 = call "PicoScopeAdcToVolts.vi"("Max_adc"=w278, "Range Index"=w299, "Data"=w276) -> ("Data"=w297:dbl[])
        n114 = call "PicoScopeAdcToVolts.vi"("Max_adc"=w278, "Range Index"=w294, "Data"=w275) -> ("Data"=w292:dbl[])
        n115 = local read "DownSample Interval (sec)"() -> (w271:dbl)
        n116 = Bundle(0, "DownSample Interval (sec)"=w271, "Data"=w298) -> (w296:T15)  [unwired: 1 in]
        n117 = Bundle(0, "DownSample Interval (sec)"=w271, "Data"=w297) -> (w295:T15)  [unwired: 1 in]
        n118 = Bundle(0, "DownSample Interval (sec)"=w271, "Data"=w292) -> (w290:T15)  [unwired: 1 in]
        n119 = Bundle(0, "DownSample Interval (sec)"=w271, "Data"=w291) -> (w289:T15)  [unwired: 1 in]
        n120 = call-poly <vilib>:"Analog to Digital.vi"("data format (offset binary)"=w287, "full-scale range (pk-pk)"=256.0, "resolution (16 bit)"=8, "analog waveform"=w270) -> ("digital waveform"=w283:digitalwaveform)  [unwired: 4 in, 3 out]
        n121 = Build Array(w296, w295, w290, w289) -> (w266:T16)
        "Analog Channels" <- w266
        n122 = Bundle By Name("t0"=timestamp(0 s since 1904-01-01), "dt"=w271, "Y"=w283) -> (→"Port 0":digitalwaveform)  [unwired: 1 in]
        n123 = case shown="True" "Write to file" {
          tunnel: w269 -> [w302 w305]
          tunnel: [w302 w304] -> w268
          tunnel: w266 -> [_ w303]
          frame False {
          }
          frame True {
            n124 = call "PicoWriteTDMS.vi"("Analog Channels"=w303, "Refnum in"=w305) -> ("Refnum out"=w304:refnum<k34>)  [unwired: 8 in, 1 out]
          }
        }
      }
    }
  }
  n125 = flat-sequence {
    tunnel: w19 -> [w313]
    tunnel: w1 -> [w312]
    tunnel: w18 -> [w311]
    tunnel: w17 -> [w310]
    tunnel: w16 -> [w320]
    tunnel: w15 -> [w319]
    tunnel: w6 -> [w318]
    tunnel: w5 -> [w317]
    tunnel: w4 -> [w316]
    tunnel: w3 -> [w315]
    frame #0 {
      n126 = call "PicoScopeospaClose.vi"("error in (no error)"=w311, "handle in"=w310) -> ("error out"=w314:errorcluster)  [unwired: 8 in, 1 out]
      n127 = call "PicoReleaseMultiBuffers.vi"("error in (no error)"=w314, "Enabled array"=w313, "Data Pointers"=w312) -> ()  [unwired: 7 in, 2 out]
    }
    frame #1 {
      n128 = Release Queue(queue=w320) -> ()  [unwired: 2 in, 3 out]
      n129 = Release Queue(queue=w319) -> ()  [unwired: 2 in, 3 out]
      n130 = Release Queue(queue=w318) -> ()  [unwired: 2 in, 3 out]
      n131 = Release Queue(queue=w317) -> ()  [unwired: 2 in, 3 out]
      n132 = Release Queue(queue=w316) -> ()  [unwired: 2 in, 3 out]
      n133 = Release Queue(queue=w315) -> ()  [unwired: 2 in, 3 out]
    }
  }
  n134 = TDMS Close(11:w26) -> ()  [unwired: 1 in, 2 out]
